vi "Waveform array size_Generated from sampling time and required time.vi"(10 "Sample time in Seconds (dT = 1/Fs)":dbl, 11 "Task time in seconds":dbl) -> (3 "Array Size OUT":i32)   [LabVIEW 2012]
doc: "This is an Inlined VI"
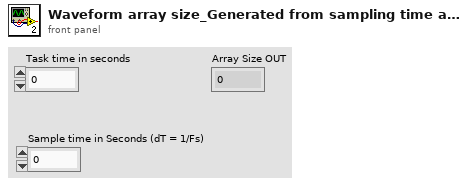
[diagram p1: front panel]
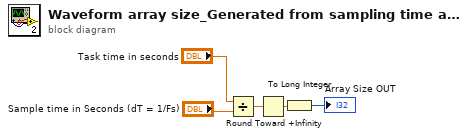
[diagram p0: block diagram]
diagram:
  n1 = Divide(x="Task time in seconds", y="Sample time in Seconds (dT = 1/Fs)") -> (x/y=w2:dbl)
  n2 = Round Toward +Infinity(x=w2) -> (ceil(x): smallest int >= x=w1:dbl)
  n3 = To Long Integer(number=w1) -> (32bit integer=→"Array Size OUT":i32)
